vi "Read Generate Signal Path.vi"(8 "error in (no error)":errorcluster, 11 "EST Knock Sensor in":refnum<class "EST Knock Sensor.lvclass">) -> (0 "error out":errorcluster, 2 "Generate Signal Path":path, 3 "EST Knock Sensor out":refnum<class "EST Knock Sensor.lvclass">)   [LabVIEW 2015, in "EST Knock Sensor.lvclass"]
uses:
  EST Knock Sensor.lvclass
  EST Knock Sensor.lvclass/EST Knock Sensor.ctl
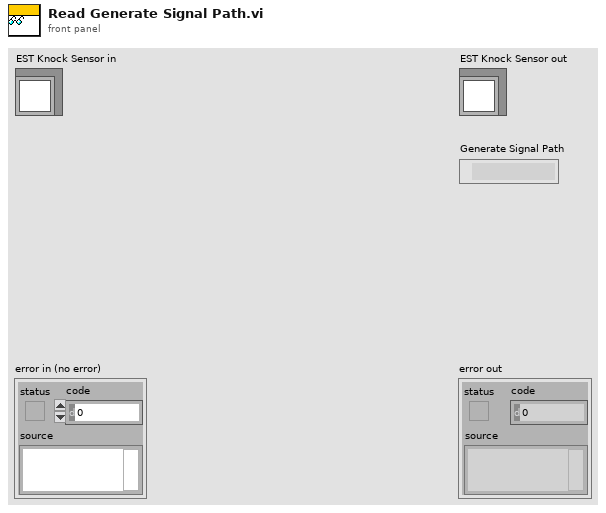
[diagram p1: front panel]
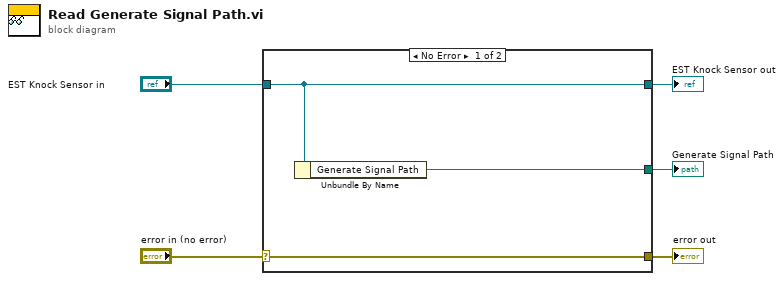
[diagram p0: block diagram]
diagram:
  n1 = case shown="No Error" "error in (no error)" {
    selector: "error in (no error)" -> [w8 w9]
    tunnel: [w8 w9] -> w4
    tunnel: [w7 w10] -> w2
    tunnel: "EST Knock Sensor in" -> [w7 w10]
    tunnel: [w6 _] -> w1
    frame No Error {
      n2 = Unbundle By Name(w7) -> ("Generate Signal Path"=w6:path)
    }
    frame Error {
    }
  }
  "error out" <- w4
  "EST Knock Sensor out" <- w2
  "Generate Signal Path" <- w1
